vi "Runtime Version.vi"(6 "error in":errorcluster) -> (0 "error out":errorcluster, 3 "Runtime Version":string, 4 "Version":T1, 5 "Local runtime":path)   [LabVIEW 2014, in "Raspberry Pi Compatible Compiler for LabVIEW.lvlib"]
uses:
  Raspberry Pi Compatible Compiler for LabVIEW.lvlib
  RasPi_Services/Download/RuntimeVersion.ctl
  GitHub/TypeDefs/GitHubCheckTypeTD.ctl
  Compile and Download App/Custom Controls/Local Setup Parameters.ctl
  GitHub/GitHub API.lvlib
  RasPi_Services/Download/RasPiDownloader.lvlib
panel:
  in  "Config File Directory":path
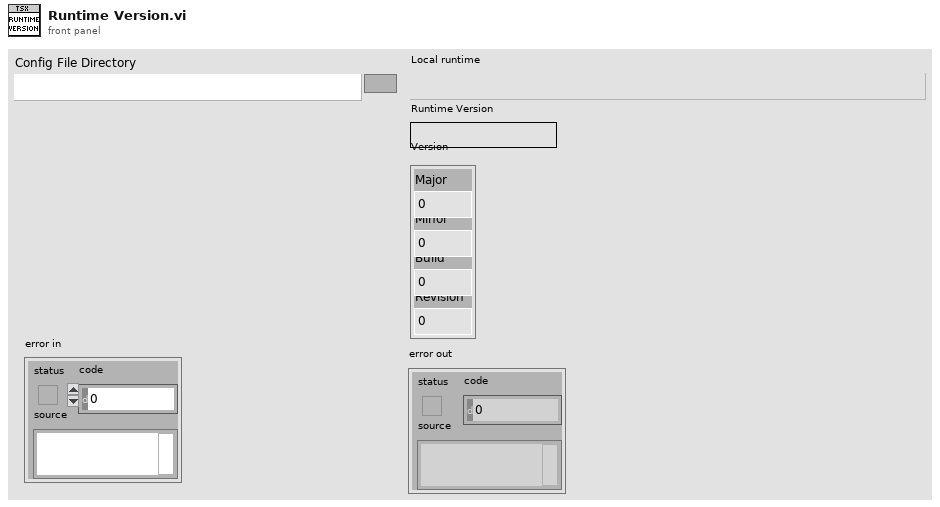
[diagram p1: front panel]
types:
  T1 = typedef "Raspberry Pi Compatible Compiler for LabVIEW.lvlib/RasPiDownloader.lvlib/RuntimeVersion.ctl" = cluster{"Major":i32, "Minor":i32, "Build":i32, "Revision":i32}
  T2 = typedef "Raspberry Pi Compatible Compiler for LabVIEW.lvlib/GitHub API.lvlib/GitHubCheckTypeTD.ctl" = enum16{"runtime", "VIPM Home Version", "VIPM Standard Version"}
  T3 = typedef "Raspberry Pi Compatible Compiler for LabVIEW.lvlib/GitHub API.lvlib/GitHubContents_TD.ctl" = cluster{"name":string, "path":string, "sha":string, "size":dbl, "url":string, "html_url":string, "git_url":string, "download_url":string, "type":string, "_links":cluster{"self":string, "git":string, "html":string}}
  T4 = typedef "Raspberry Pi Compatible Compiler for LabVIEW.lvlib/Local Setup Parameters.ctl" = enum16{"Add Last VI", "Read Last VI", "Add Board IP", "Remove Board IP", "Read All Board IP", "Add Runtime Version", "Read Runtime Version", "Add Package Version", "Read Package Version", "Add VIPCheck Time", "Read VIPCheck Time"}
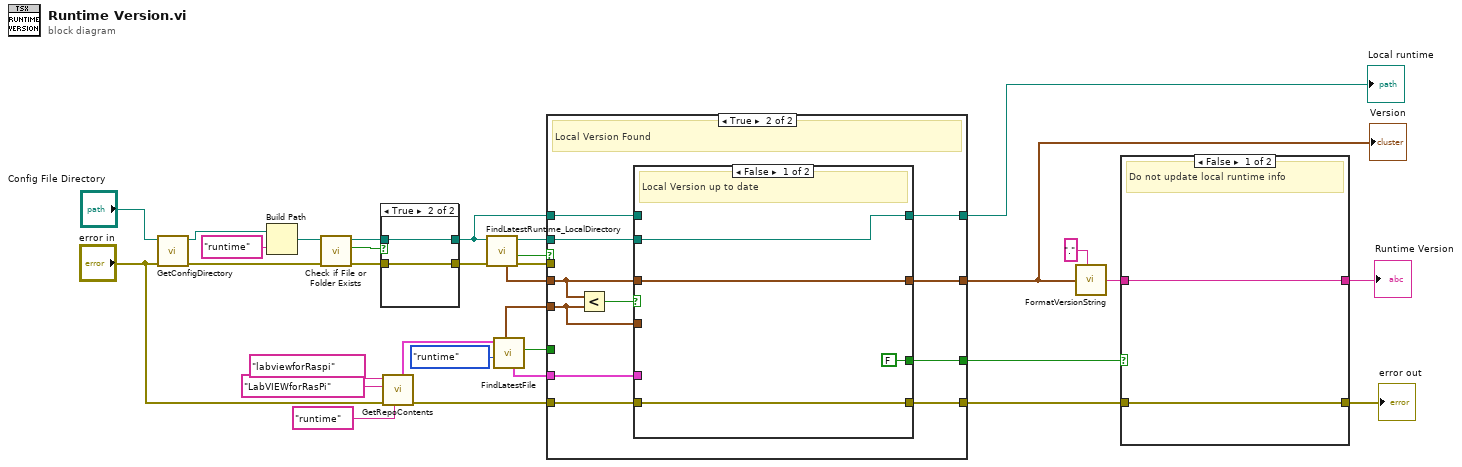
[diagram p0: block diagram]
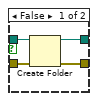
[diagram p2: hidden frame]
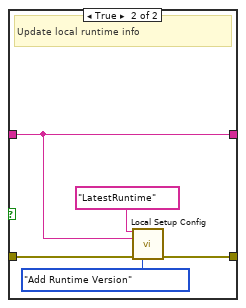
[diagram p3: hidden frame]
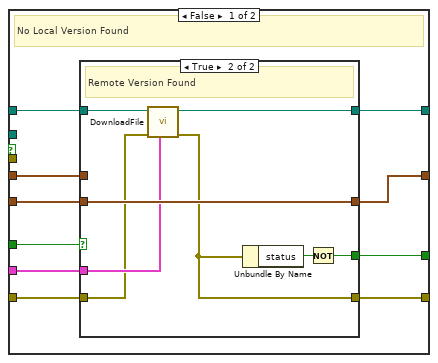
[diagram p4: hidden frame]
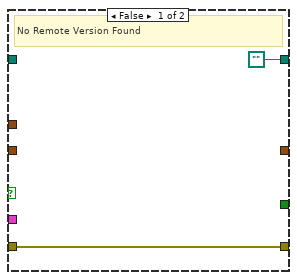
[diagram p5: hidden frame]
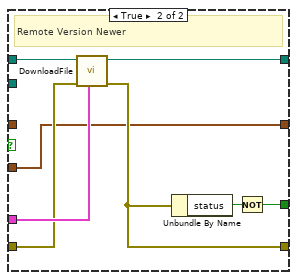
[diagram p6: hidden frame]
diagram:
  n1 = call "GetConfigDirectory.vi"("error in"="error in", "Config File Directory"="Config File Directory") -> ("error out"=w7:errorcluster, "config file directory out"=w3:path)  [unwired: 8 in]
  n2 = Build Path(base path=w3, name or relative path="runtime") -> (appended path=w2:path)
  n3 = call <vilib>:"Check if File or Folder Exists.vi"("error in (no error)"=w7, "path"=w2) -> ("error out"=w6:errorcluster, "file or folder exists?"=w8:bool, "dup path"=w9:path)  [unwired: 7 in]
  n4 = case shown="True" w8 {
    tunnel: [w36 w38] -> w4
    tunnel: w9 -> [w35 w38]
    tunnel: w6 -> [w34 w37]
    tunnel: [w33 w37] -> w5
    frame False {
      n5 = Create Folder(path (use dialog)=w35, error in=w34) -> (created path=w36:path, error out=w33:errorcluster)  [unwired: 1 in, 1 out]
    }
    frame True {
    }
  }
  n6 = call "GetRepoContents.vi"("path"="runtime", "error in"="error in", "repo"="LabVIEWforRasPi", "owner"="labviewforRaspi") -> ("error out"=w22:errorcluster, "Contents"=w31:T3[])  [unwired: 4 in]
  n7 = call "FindLatestRuntime_LocalDirectory.vi"("error in"=w5, "Path"=w4) -> ("error out"=w21:errorcluster, "Found"=w27:bool, "local runtime path"=w12:path, "Version"=w25:T1)  [unwired: 4 in]
  n8 = call "FindLatestFile.vi"("Check Type"=GitHubCheckTypeTD."runtime", "Contents"=w31) -> ("Found"=w26:bool, "Latest runtime"=w23:T3, "Version"=w24:T1)  [unwired: 5 in]
  n9 = case shown="True" w27 {
    tunnel: w26 -> [w48 _]
    tunnel: w25 -> [w47 w61]
    tunnel: w24 -> [w46 w63]
    tunnel: w23 -> [w45 w67]
    tunnel: w22 -> [w44 w68]
    tunnel: [w43 w62] -> w15
    tunnel: w4 -> [w40 w66]
    tunnel: [w42 w64] -> w19
    tunnel: [w41 w65] -> w20
    tunnel: w21 -> [_ _]
    tunnel: [w39 w60] -> w11
    tunnel: w12 -> [_ w59]
    frame False {
      # "No Local Version Found"
      n10 = case shown="True" w48 {
        tunnel: w47 -> [_ _]
        tunnel: w46 -> [_ w58]
        tunnel: w45 -> [_ w57]
        tunnel: w44 -> [w50 w56]
        tunnel: [_ w58] -> w43
        tunnel: [w50 w55] -> w42
        tunnel: [_ w53] -> w41
        tunnel: w40 -> [_ w52]
        tunnel: [path "" w51] -> w39
        frame False {
          # "No Remote Version Found"
        }
        frame True {
          # "Remote Version Found"
          n11 = call "DownloadFile.vi"("Latest runtime"=w57, "error in"=w56, "Download Folder"=w52) -> ("error out"=w55:errorcluster, "file"=w51:path)  [unwired: 5 in]
          n12 = Unbundle By Name(w55) -> ("status"=w54:bool)
          n13 = Not(x=w54) -> (.not. x?=w53:bool)
        }
      }
    }
    frame True {
      # "Local Version Found"
      n14 = Less?(x=w61, y=w63) -> (x < y?=w69:bool)
      n15 = case shown="False" w69 {
        tunnel: w67 -> [_ w80]
        tunnel: w68 -> [w71 w79]
        tunnel: [w73 w75] -> w62
        tunnel: w66 -> [_ w81]
        tunnel: [w71 w78] -> w64
        tunnel: [FALSE w76] -> w65
        tunnel: w63 -> [_ w75]
        tunnel: w61 -> [w73 _]
        tunnel: [w70 w74] -> w60
        tunnel: w59 -> [w70 _]
        frame False {
          # "Local Version up to date"
        }
        frame True {
          # "Remote Version Newer"
          n16 = call "DownloadFile.vi"("Latest runtime"=w80, "error in"=w79, "Download Folder"=w81) -> ("error out"=w78:errorcluster, "file"=w74:path)  [unwired: 5 in]
          n17 = Unbundle By Name(w78) -> ("status"=w77:bool)
          n18 = Not(x=w77) -> (.not. x?=w76:bool)
        }
      }
    }
  }
  "Local runtime" <- w11
  "Version" <- w15
  n19 = call "FormatVersionString.vi"("Version"=w15, "delimiter"=".") -> ("Version string"=w14:string)  [unwired: 1 in]
  n20 = case shown="False" w20 {
    tunnel: w19 -> [w82 w87]
    tunnel: [w82 w86] -> w17
    tunnel: [w83 w84] -> w18
    tunnel: w14 -> [w83 w84]
    frame False {
      # "Do not update local runtime info"
    }
    frame True {
      # "Update local runtime info"
      n21 = call "Local Setup Config.vi"("KeyName"="LatestRuntime", "Local Setup Param"=Local_Setup_Parameters."Add Runtime Version", "KeyValue"=w84, "error in"=w87) -> ("error out"=w86:errorcluster)  [unwired: 8 in, 3 out]
    }
  }
  "Runtime Version" <- w18
  "error out" <- w17
